vi "Write configured channels.vi"(8 "error in (no error)":errorcluster, 10 "configured channels":refnum<class "TBM channel.lvclass">[](array[class]), 11 "control module configuration in":refnum<class "control module configuration.lvclass">) -> (0 "error out":errorcluster, 3 "control module configuration out":refnum<class "control module configuration.lvclass">)   [LabVIEW 2013, in "control module configuration.lvclass"]
uses:
  control module configuration.lvclass
  <vilib>/NI/Tag Bus Module Framework/channel/TBM channel.lvclass
  control module configuration.lvclass/control module configuration.ctl
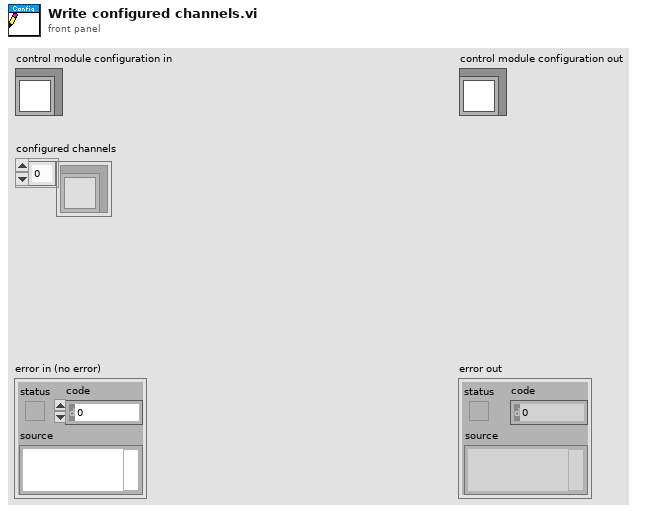
[diagram p1: front panel]
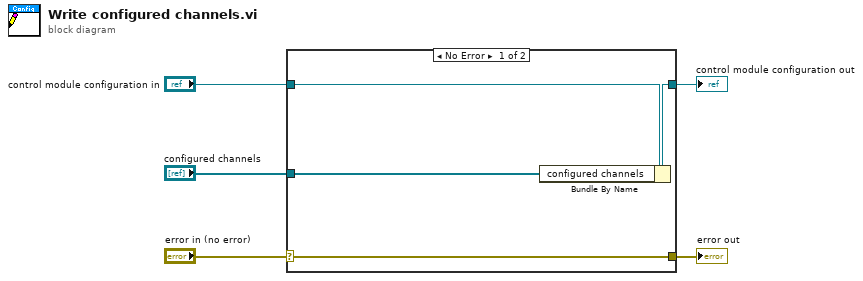
[diagram p0: block diagram]
diagram:
  n1 = case shown="No Error" "error in (no error)" {
    selector: "error in (no error)" -> [w9 w10]
    tunnel: [w9 w10] -> w4
    tunnel: [w7 w11] -> w2
    tunnel: "control module configuration in" -> [w8 w11]
    tunnel: "configured channels" -> [w6 _]
    frame No Error {
      n2 = Bundle By Name(cluster=w8, "configured channels"=w6) -> (w7:refnum<class "control module configuration.lvclass">)
    }
    frame Error {
    }
  }
  "error out" <- w4
  "control module configuration out" <- w2
